vi "Wait Till End of Processing Status.vi"(6 "Loop Timeout (ms) (5000)":i32=5000, 8 "error in (no error)":errorcluster) -> (0 "error out":errorcluster, 3 "Last Status":T1)   [LabVIEW 2019, in "ACSVcontrol-driver.lvlib"]
doc: "This VI waits till status of the PJVS is something different than \"processing\" or error appears or abort signal happens or timeout happens.\nCheck loop is at least 150 ms long."
uses:
  ACSVcontrol-driver.lvlib
  Type definitions/Status.ctl
  <vilib>/Utility/error.llb/Error Cluster From Error Code.vi
  <vilib>/ErrorRing/Error Ring.xnode
panel:
  out "Actual Status":T1
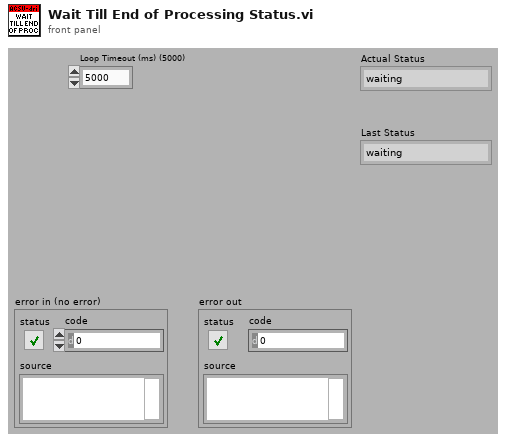
[diagram p1: front panel]
types:
  T1 = typedef "ACSVcontrol-driver.lvlib/Status.ctl" = enum16{"waiting", "processing", "error command", "Set_PJVS-Done", "Set_Mux-Done", "Set_Mux-Error", "Set_57XX-Done", "Set_57XX-Error", "Set_Gen-Done", "Set_Gen-Error", "Set_Synthesizer-Done", "Set_Synthesizer-Error", "Read_Nano-Done", "Read_Sampler-Done", "Read_Sampler-Error", "Read_Sensors-Done"}
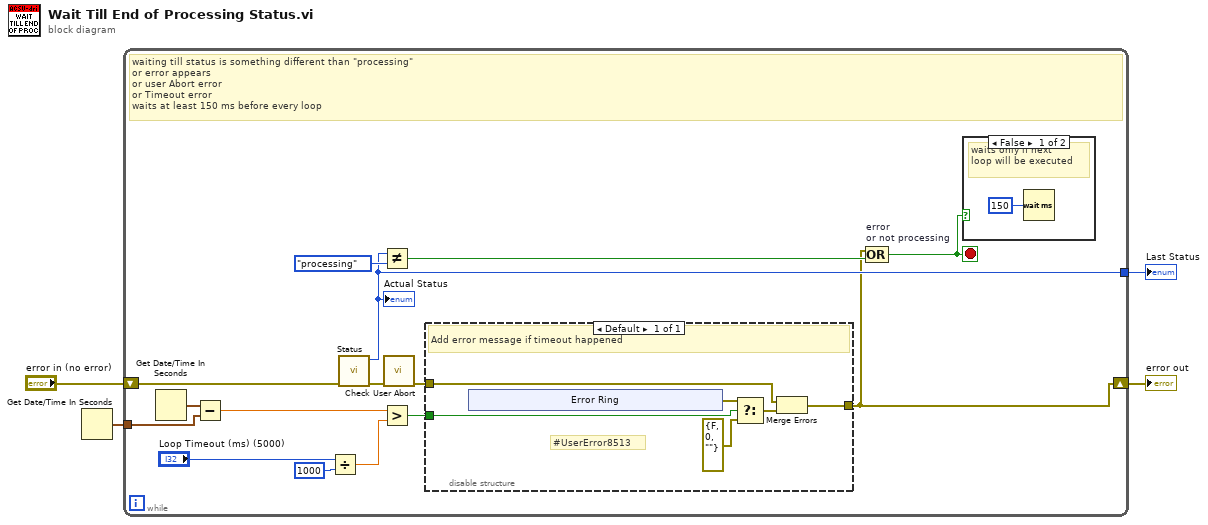
[diagram p0: block diagram]
diagram:
  n1 = Get Date/Time In Seconds() -> (seconds since 1Jan1904=w2:timestamp)
  n2 = while {
    shift-right: [w6] -> w4
    shift-left: "error in (no error)" -> [w14]
    tunnel: w2 -> [w17]
    tunnel: [w13] -> w1
    stop <- w5 stop-if-true
    # "waiting till status is something different than \"processing\"\nor error appears\nor user Abort error \nor Timeout error\nwaits at least 150 ms before every loop"
    n3 = Get Date/Time In Seconds() -> (seconds since 1Jan1904=w16:timestamp)
    n4 = Subtract(x=w16, y=w17) -> (x-y=w15:dbl)
    n5 = Divide(x="Loop Timeout (ms) (5000)", y=1000) -> (x/y=w11:dbl)
    n6 = call "Status.vi"("error in (no error)"=w14) -> ("error out"=w8:errorcluster, "Status"=w13:T1)  [unwired: 7 in, 2 out]
    "Actual Status" <- w13
    n7 = Not Equal?(x=w13, y=Status."processing" ("x")) -> (x != y?=w18:bool)
    n8 = Greater?(x=w15, y=w11) -> (0:w9:bool)
    n9 = call "Check User Abort.vi"("error in (no error)"=w8) -> ("error out"=w7:errorcluster)  [unwired: 10 in]
    n10 = disable-structure shown="Default" {
      disable-tunnel: w7 -> [w26]
      disable-tunnel: w9 -> [w23]
      disable-tunnel: [w21] -> w6
      frame Enabled {
        # "#UserError8513"
        # "Add error message if timeout happened"
        n11 = xnode "Error Ring"() -> ("error out"=w24:errorcluster)
        n12 = Select(t=w24, s=w23, f=errorcluster {"status"=FALSE, "code"=0, "source"=""}) -> (s? t:f=w25:errorcluster)
        n13 = Merge Errors(w26, w25) -> (w21:errorcluster)
      }
    }
    n14 = Compound Arithmetic op=OR "error\nor not processing"(w6, w18) -> (w5:bool)
    n15 = case shown="False" w5 {
      frame False {
        # "waits only if next\nloop will be executed"
        n16 = Wait (ms)(milliseconds to wait=u32 150) -> ()  [unwired: 1 out]
      }
      frame True {
      }
    }
  }
  "error out" <- w4
  "Last Status" <- w1
